vi "Set Window Position.vi"(0 "X":i32, 5 "Hwnd":u32, 7 "Y":i32, 9 "Width":i32, 11 "error in (no error)":errorcluster, 12 "Height":i32) -> (15 "error out":errorcluster)   [LabVIEW 2019, in "LV MDI.lvclass"]
doc: "Set window bounds to specified window."
uses:
  LV MDI.lvclass
  user32.dll
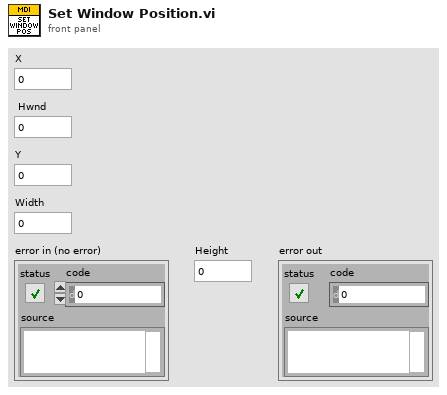
[diagram p1: front panel]
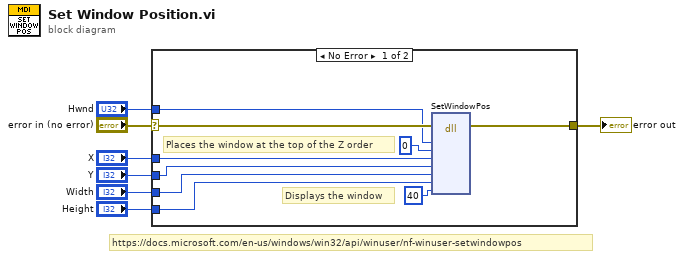
[diagram p0: block diagram]
diagram:
  # "https://docs.microsoft.com/en-us/windows/win32/api/winuser/nf-winuser-setwindowpos"
  n1 = case shown="No Error" "error in (no error)" {
    selector: "error in (no error)" -> [w11 w17]
    tunnel: [w16 w17] -> w7
    tunnel: "X" -> [w15 _]
    tunnel: "Y" -> [w14 _]
    tunnel: "Height" -> [w13 _]
    tunnel: "Width" -> [w12 _]
    tunnel: "Hwnd" -> [w10 _]
    frame No Error {
      # "Displays the window"
      # "Places the window at the top of the Z order"
      n2 = dll-call lib="user32.dll" fn="SetWindowPos"(error in=w11, "Hwnd"=w10, "hwndInsertafter"=0, "x"=w15, "y"=w14, "cx"=w12, "cy"=w13, "uflags"=40) -> (error out=w16:errorcluster)  [unwired: 10 in, 1 out]
    }
    frame Error {
    }
  }
  "error out" <- w7
